vi "Expanded Terminal Bounds.vi"(8 "Header":i32, 9 "Input":bool, 10 "Border Without Terminals":T1, 11 "Index":i32) -> (3 "Bounds":T2)   [LabVIEW 2020, in "Parallel Diagram Block.xnode"]
uses:
  Parallel Diagram Block.xnode
  <vilib>/XNodeSupport/XNodeInt.ctl
  <vilib>/XNodeSupport/NI_XNodeSupport.lvlib
  <vilib>/XNodeSupport/XNodeRect32.ctl
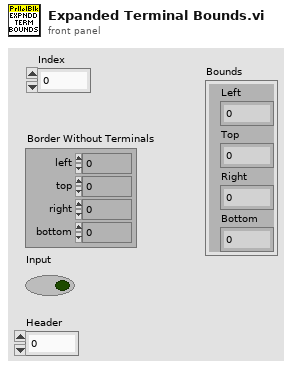
[diagram p1: front panel]
types:
  T1 = cluster{"left":i16, "top":i16, "right":i16, "bottom":i16}
  T2 = typedef "NI_XNodeSupport.lvlib/XNodeRect32.ctl" = cluster{"Left":T3, "Top":T3, "Right":T3, "Bottom":T3}
  T3 = typedef "NI_XNodeSupport.lvlib/XNodeInt.ctl" = i32
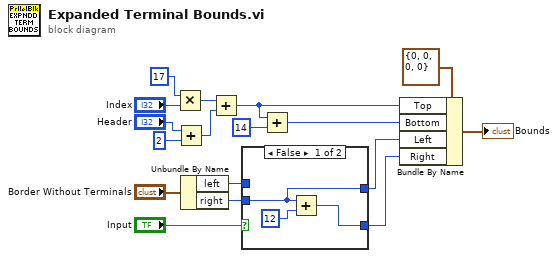
[diagram p0: block diagram]
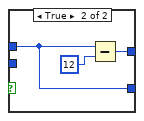
[diagram p2: hidden frame]
diagram:
  n1 = Multiply(x=17 ("y"), y="Index") -> (x*y=w15:i32)
  n2 = Add(x="Header", y=2) -> (x+y=w2:i32)
  n3 = Unbundle By Name("Border Without Terminals") -> ("left"=w5:i16, "right"=w6:i16)
  n4 = Add(x=w15, y=w2) -> (x+y=w11:i32)
  n5 = case shown="False" "Input" {
    tunnel: w6 -> [w20 _]
    tunnel: w5 -> [_ w21]
    tunnel: [w20 w22] -> w4
    tunnel: [w18 w21] -> w3
    frame False {
      n6 = Add(x=w20, y=i16 12) -> (x+y=w18:i16)
    }
    frame True {
      n7 = Subtract(x=w21, y=i16 12) -> (x-y=w22:i16)
    }
  }
  n8 = Add(x=w11, y=14) -> (x+y=w9:i32)
  n9 = Bundle By Name(cluster=T2 {"Left"=0, "Top"=0, "Right"=0, "Bottom"=0} ("Bounds"), "Top"=w11, "Bottom"=w9, "Left"=w4, "Right"=w3) -> (→"Bounds":T2)
